vi "Atan2 to +-Pi Scale.vi"(1 "atan2 result":dbl) -> (0 "Scaled":dbl)   [LabVIEW 2016]
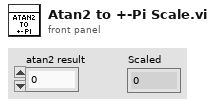
[diagram p1: front panel]
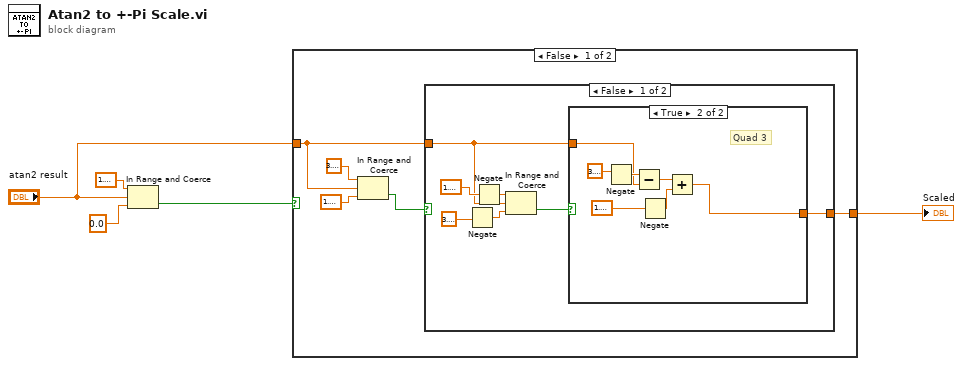
[diagram p0: block diagram]
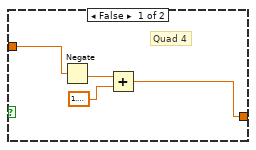
[diagram p2: hidden frame]
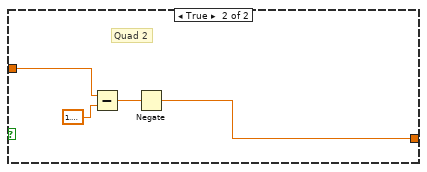
[diagram p3: hidden frame]
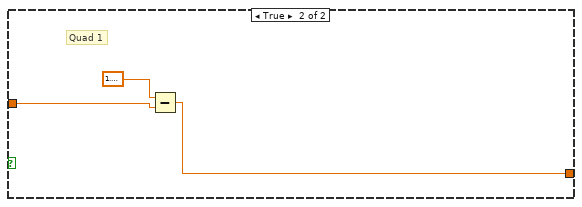
[diagram p4: hidden frame]
diagram:
  n1 = In Range and Coerce(upper limit=1.5707963267948966, x="atan2 result", lower limit=0.0) -> (In Range?=w3:bool)  [unwired: 1 out]
  n2 = case shown="False" w3 {
    tunnel: "atan2 result" -> [w7 w34]
    tunnel: [w6 w33] -> w1
    frame False {
      n3 = In Range and Coerce(upper limit=3.141592653589793, x=w7, lower limit=1.5707963267948966) -> (In Range?=w8:bool)  [unwired: 1 out]
      n4 = case shown="False" w8 {
        tunnel: w7 -> [w12 w32]
        tunnel: [w11 w29] -> w6
        frame False {
          n5 = Negate(x=3.141592653589793) -> (-x=w13:dbl)
          n6 = Negate(x=1.5707963267948966) -> (-x=w16:dbl)
          n7 = In Range and Coerce(upper limit=w16, x=w12, lower limit=w13) -> (In Range?=w17:bool)  [unwired: 1 out]
          n8 = case shown="True" w17 {
            tunnel: w12 -> [w21 w26]
            tunnel: [w18 w22] -> w11
            frame False {
              # "Quad 4"
              n9 = Negate(x=w21) -> (-x=w20:dbl)
              n10 = Add(x=w20, y=1.5707963267948966) -> (x+y=w18:dbl)
            }
            frame True {
              # "Quad 3"
              n11 = Negate(x=3.141592653589793) -> (-x=w27:dbl)
              n12 = Subtract(x=w27, y=w26) -> (x-y=w25:dbl)
              n13 = Negate(x=1.5707963267948966) -> (-x=w23:dbl)
              n14 = Add(x=w25, y=w23) -> (x+y=w22:dbl)
            }
          }
        }
        frame True {
          # "Quad 2"
          n15 = Subtract(x=w32, y=1.5707963267948966) -> (x-y=w30:dbl)
          n16 = Negate(x=w30) -> (-x=w29:dbl)
        }
      }
    }
    frame True {
      # "Quad 1"
      n17 = Subtract(x=1.5707963267948966, y=w34) -> (x-y=w33:dbl)
    }
  }
  "Scaled" <- w1
